vi "Configure Arbitrary Waveform.vi"(6 "DC Offset (0 V)":dbl, 7 "Waveform Data":dbl[](array[numeric]), 8 "error in (no error)":errorcluster, 9 "Frequency (100000 Hz)":dbl=100000.0, 10 "Amplitude (0.5 V)":dbl=0.5, 11 "VISA resource name":refnum<visa-resource-name>) -> (0 "error out":errorcluster, 3 "VISA resource name out":refnum<visa-resource-name>)   [LabVIEW 2017, in "Scope.lvlib" / "Tektronix DPO MSO 2000 4000 Series.lvlib"]
doc: "Configures the arbitrary waveform.\n\n<B>Notes:</B>\n(1) This VI is available for MDO3000 Series only.\n\n(2) Requires the MDO3AFG option to be installed."
uses:
  Tektronix DPO MSO 2000 4000 Series.lvlib
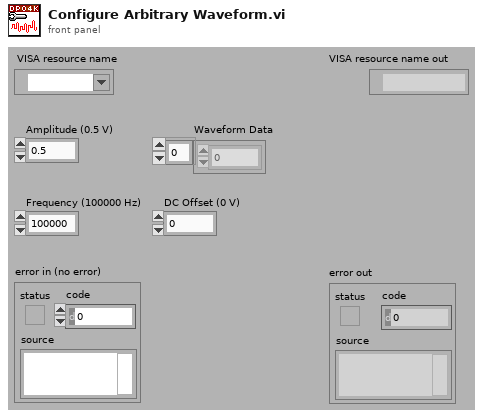
[diagram p1: front panel]
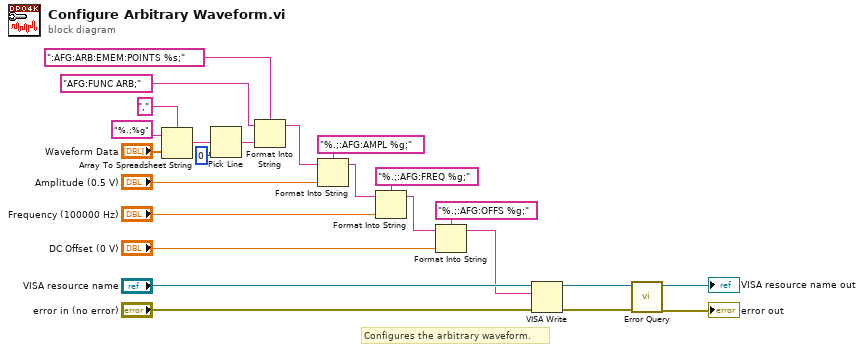
[diagram p0: block diagram]
diagram:
  # "Configures the arbitrary waveform."
  n1 = Array To Spreadsheet String(delimiter (Tab)=",", array="Waveform Data", 3:"%.;%g" ("format string")) -> (spreadsheet string=w4:string)
  n2 = Pick Line(multi-line string=w4, line index=0) -> (output string=w3:string)  [unwired: 1 in]
  n3 = Format Into String(format string=":AFG:ARB:EMEM:POINTS %s;", initial string="AFG:FUNC ARB;", w3) -> (resulting string=w5:string)  [unwired: 1 in, 1 out]
  n4 = Format Into String(format string="%.;:AFG:AMPL %g;", initial string=w5, "Amplitude (0.5 V)") -> (resulting string=w7:string)  [unwired: 1 in, 1 out]
  n5 = Format Into String(format string="%.;:AFG:FREQ %g;", initial string=w7, "Frequency (100000 Hz)") -> (resulting string=w8:string)  [unwired: 1 in, 1 out]
  n6 = Format Into String(format string="%.;:AFG:OFFS %g;", initial string=w8, "DC Offset (0 V)") -> (resulting string=w6:string)  [unwired: 1 in, 1 out]
  n7 = VISA Write(VISA resource name="VISA resource name", write buffer=w6, error in (no error)="error in (no error)") -> (VISA resource name out=w17:refnum<visa-resource-name>, error out=w16:errorcluster)  [unwired: 1 out]
  n8 = call "Error Query.vi"("error in (no error)"=w16, "VISA resource name"=w17) -> ("error out"=→"error out":errorcluster, "VISA resource name out"=→"VISA resource name out":refnum<visa-resource-name>)  [unwired: 6 in, 2 out]
